vi "Run IV Curve Plugin.vi"   [LabVIEW 2019]
uses:
  MeasurementSMO/MeasurementSMO.lvclass
  <vilib>/JKI/JKI SMO/SMO/SMO.lvclass
  C:/Program Files (x86)/National Instruments/LabVIEW 2019/vi.lib/JKI/JKI SMO/SMO/SMO.lvclass
types:
  T1 = typedef "SMO.lvclass/Public Events.ctl" = cluster{"Error":refnum<user-event>, "State":refnum<user-event>, "Reserve State":refnum<user-event>}
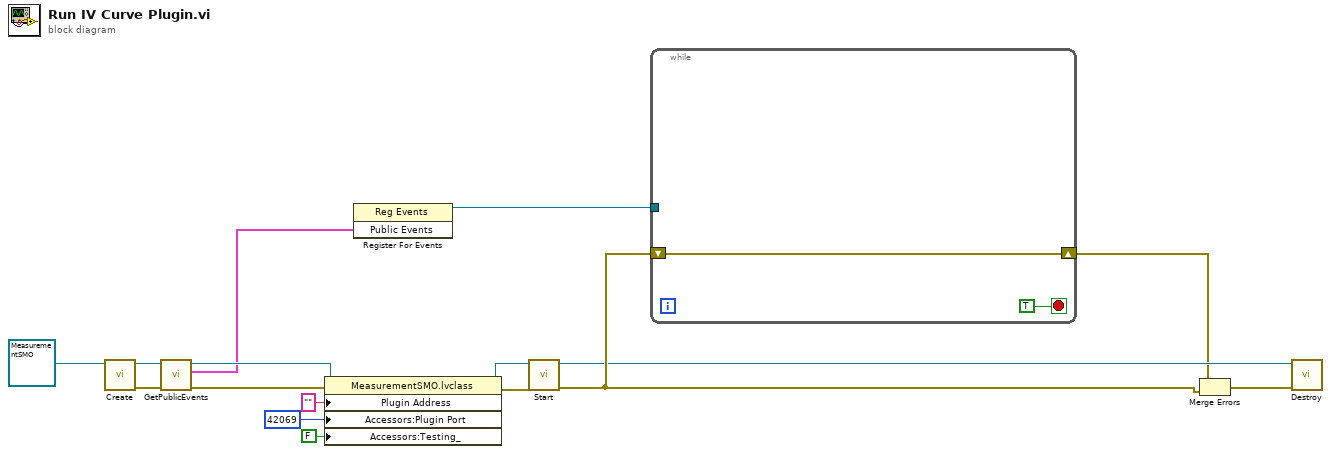
[diagram p0: block diagram]
diagram:
  n1 = call <vilib>:"Create.vi"("SMO"=refnum<class "MeasurementSMO.lvclass"> refnum ("MeasurementSMO.lvclass")) -> ("error out"=w7:errorcluster, "SMO out"=w12:refnum<class "MeasurementSMO.lvclass">)  [unwired: 8 in, 1 out]
  n2 = call <vilib>:"GetPublicEvents.vi"("error in (no error)"=w7, "SMO"=w12) -> ("error out"=w15:errorcluster, "Public Events"=w6:T1, "SMO out"=w16:refnum<class "MeasurementSMO.lvclass">)  [unwired: 7 in]
  n3 = property class="MeasurementSMO.lvclass"(reference=w16, error in=w15, "Plugin Address"="", "Accessors:Plugin Port"=u16 42069 ("Plugin Port"), "Accessors:Testing_"=FALSE ("Testing_")) -> (reference out=w14:refnum<class "MeasurementSMO.lvclass">, error out=w11:errorcluster)
  n4 = register-events(w6) -> (reference out=w5:refnum<event-registration>)  [unwired: 2 in, 1 out]
  n5 = call <vilib>:"Start.vi"("error in (no error)"=w11, "SMO"=w14) -> ("error out"=w4:errorcluster, "SMO out"=w3:refnum<class "MeasurementSMO.lvclass">)  [unwired: 8 in]
  n6 = while {
    tunnel: w5 -> [_]
    shift-right: [w18] -> w1
    shift-left: w4 -> [w18]
    stop <- TRUE stop-if-true
  }
  n7 = Merge Errors(w1, w4) -> (w2:errorcluster)
  n8 = call <vilib>:"Destroy.vi"("error in (no error)"=w2, "SMO"=w3) -> ()  [unwired: 9 in, 1 out]
